vi "Save.vi"(8 "error in (no error)":errorcluster, 9 "new command":string, 10 "Msg in":T1, 11 "FakePressureController in":refnum<class "MagAnalysis_Online.lvclass">) -> (0 "error out":errorcluster, 1 "Path":path, 2 "Msg out":T1, 3 "FakePressureController out":refnum<class "MagAnalysis_Online.lvclass">, 4 "new command":string)   [LabVIEW 2011, in "MagAnalysis_Online.lvclass"]
uses:
  MagAnalysis_Online.lvclass
  DriverMsg.ctl
  MagAnalysis_Online.lvclass/MagAnalysis_Online.ctl
  DaqPad_NI6009.lvclass
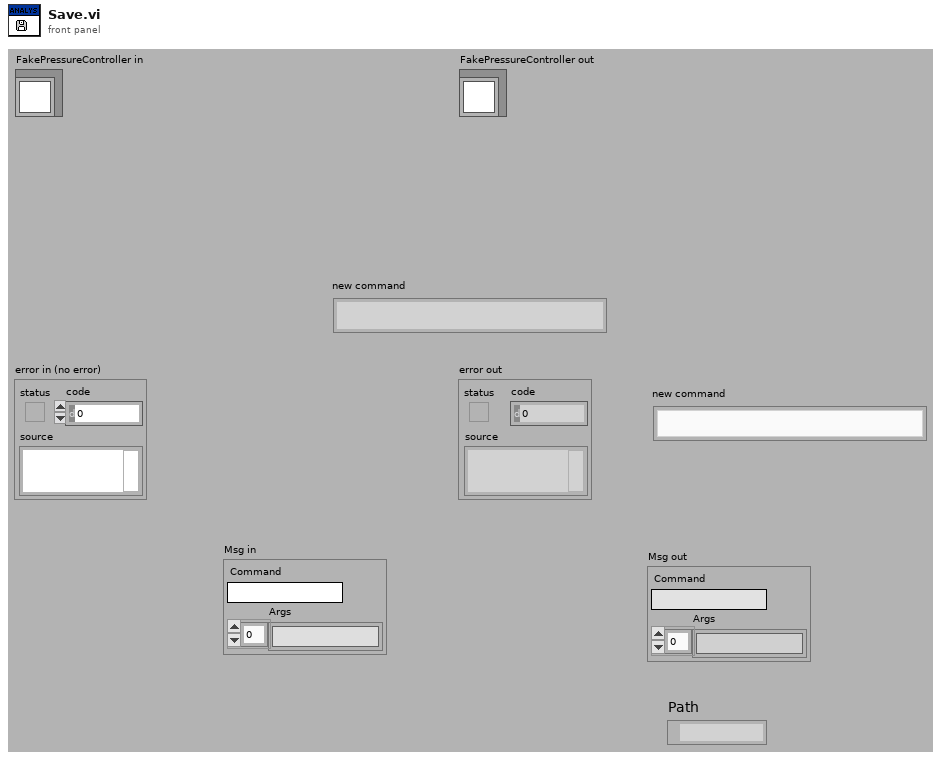
[diagram p1: front panel]
types:
  T1 = typedef "DriverMsg.ctl" = cluster{"Command":string, "Args":string[]}
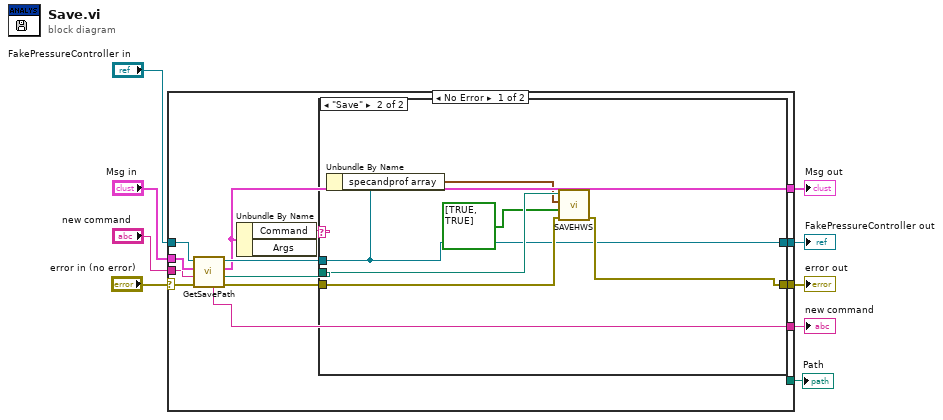
[diagram p0: block diagram]
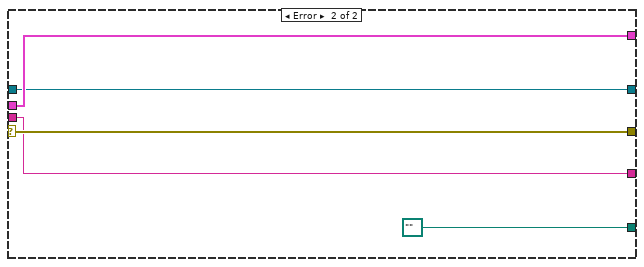
[diagram p3: hidden frame]
diagram:
  n1 = case shown="No Error" "error in (no error)" {
    selector: "error in (no error)" -> [w15 w34]
    tunnel: [w19 w34] -> w5
    tunnel: [_ path "" ("Path")] -> w1
    tunnel: [w13 w33] -> w6
    tunnel: [w20 w32] -> w8
    tunnel: "Msg in" -> [w17 w33]
    tunnel: "FakePressureController in" -> [w18 w32]
    tunnel: "new command" -> [w16 w30]
    tunnel: [w10 w30] -> w2
    frame No Error {
      n2 = call-dynamic "GetSavePath.vi"("error in (no error)"=w15, "new command"=w16, "Msg in"=w17, "BaseDriver in"=w18) -> ("error out"=w11:errorcluster, "Path"=w12:path, "Msg out"=w13:T1, "BaseDriver out"=w14:refnum<class "MagAnalysis_Online.lvclass">, "new command"=w10:string)  [unwired: 3 in]
      n3 = Unbundle By Name(w13) -> ("Command"=w21:string)  [unwired: 1 out]
      n4 = case shown="\"Save\"" w21 {
        tunnel: w14 -> [w23 w25]
        tunnel: [w23 w25] -> w20
        tunnel: w12 -> [_ w29]
        tunnel: w11 -> [w22 w27]
        tunnel: [w22 w26] -> w19
        frame Default {
        }
        frame "Save" {
          n5 = Unbundle By Name(w25) -> ("specandprof array"=w24:waveform(dbl)[])
          n6 = call "SAVEHWS.vi"("error in (no error)"=w27, "Enable (Array)"=bool[] [TRUE, TRUE], "data"=w24, "Destination HWS File"=w29) -> ("error out"=w26:errorcluster)  [unwired: 7 in]
        }
      }
    }
    frame Error {
    }
  }
  "error out" <- w5
  "FakePressureController out" <- w8
  "Path" <- w1
  "Msg out" <- w6
  "new command" <- w2
